vi "MongoDB.DocumentUpdate.vi"(8 "error in (no error)":errorcluster, 11 "MongoDB.Collection in":refnum<class "MongoDB.Collection.lvclass">) -> (0 "error out":errorcluster, 2 "Result":T1, 3 "MongoDB.Collection out":refnum<class "MongoDB.Collection.lvclass">)   [LabVIEW 2014, in "MongoDB.Collection.lvclass"]
uses:
  MongoDB.Collection.lvclass
  C:/Users/Richard/Documents/GitHub/mongo-labview-driver/CSharp/bin/MongoDB.Driver.Core.dll
  CSharp/bin/MongoDB.Driver.Core.dll
  C:/Users/Richard/Documents/GitHub/mongo-labview-driver/CSharp/bin/MongoDB.Bson.dll
  CSharp/bin/MongoDB.Bson.dll
  C:/Users/Richard/Documents/GitHub/mongo-labview-driver/CSharp/bin/MongoDB.Driver.Legacy.dll
  CSharp/bin/MongoDB.Driver.Legacy.dll
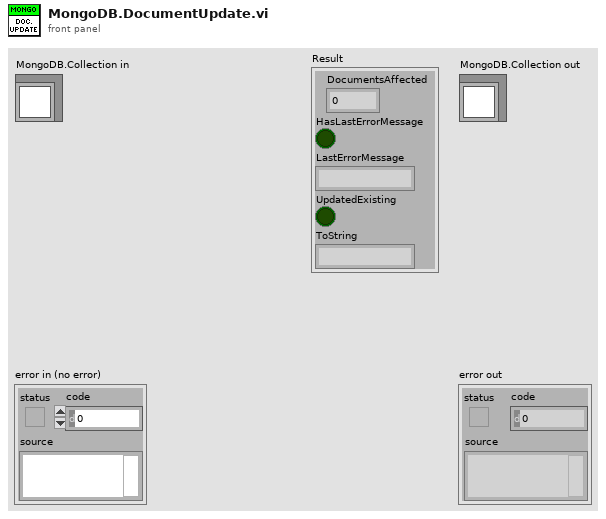
[diagram p1: front panel]
types:
  T1 = cluster{"DocumentsAffected":i64, "HasLastErrorMessage":bool, "LastErrorMessage":string, "UpdatedExisting":bool, "ToString":string}
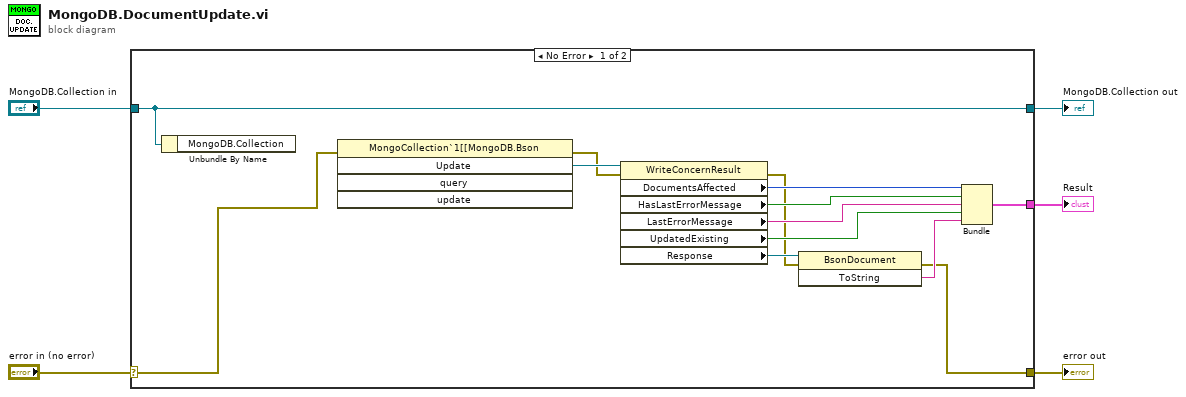
[diagram p0: block diagram]
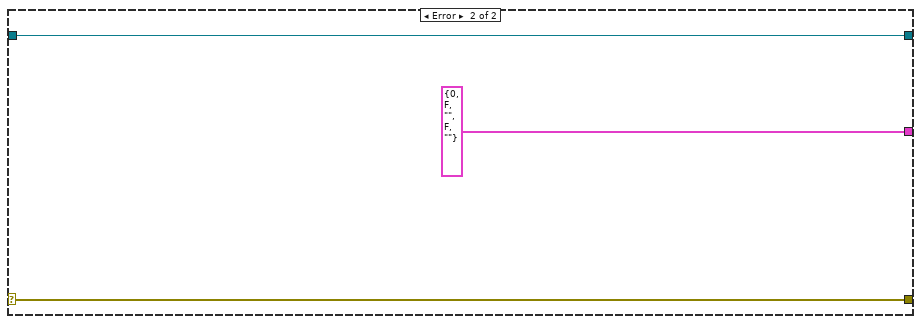
[diagram p2: hidden frame]
diagram:
  n1 = case shown="No Error" "error in (no error)" {
    selector: "error in (no error)" -> [w6 w21]
    tunnel: [w8 w21] -> w4
    tunnel: [w18 w20] -> w2
    tunnel: "MongoDB.Collection in" -> [w18 w20]
    tunnel: [w7 T1 {"DocumentsAffected"=0, "HasLastErrorMessage"=FALSE, "LastErrorMessage"="", "UpdatedExisting"=FALSE, "ToString"=""}] -> w1
    frame No Error {
      n2 = Unbundle By Name(w18) -> ()  [unwired: 1 out]
      n3 = invoke class="MongoCollection`1[[MongoDB.Bson" method="Update"(error in=w6) -> (error out=w16:errorcluster, "Update"=w17:refnum<k24>)  [unwired: 4 in, 3 out]
      n4 = property class="WriteConcernResult"(reference=w17, error in=w16) -> (error out=w9:errorcluster, "DocumentsAffected"=w15:i64, "HasLastErrorMessage"=w14:bool, "LastErrorMessage"=w13:string, "UpdatedExisting"=w12:bool, "Response"=w11:refnum<k24>)  [unwired: 1 out]
      n5 = invoke class="BsonDocument" method="ToString"(reference=w11, error in=w9) -> (error out=w8:errorcluster, "ToString"=w10:string)  [unwired: 1 in, 1 out]
      n6 = Bundle("DocumentsAffected"=w15, "HasLastErrorMessage"=w14, "LastErrorMessage"=w13, "UpdatedExisting"=w12, "ToString"=w10) -> (w7:T1)  [unwired: 1 in]
    }
    frame Error {
    }
  }
  "error out" <- w4
  "MongoDB.Collection out" <- w2
  "Result" <- w1
